vi "RSZVB Get Remote Display Title.vi"(8 "error in (no error)":errorcluster {"code" format="%.0x"}, 11 "VISA session":refnum<visa-resource-name>) -> (0 "error out":errorcluster {"code" format="%.0x"}, 1 "Title":string, 3 "dup VISA session":refnum<visa-resource-name>)   [LabVIEW 2011]
doc: "This function queries title for the remote display.\n\nRemote-control command(s):\nSYSTem:USER:DISPlay:TITLe?"
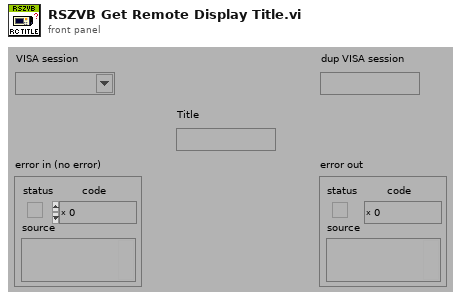
[diagram p1: front panel]
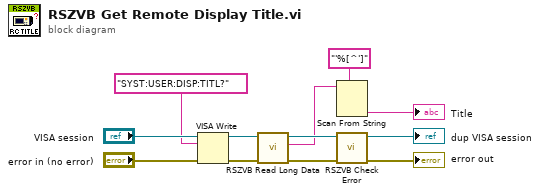
[diagram p0: block diagram]
diagram:
  n1 = VISA Write(VISA resource name="VISA session", write buffer="SYST:USER:DISP:TITL?", error in (no error)="error in (no error)") -> (VISA resource name out=w5:refnum<visa-resource-name>, error out=w4:errorcluster)  [unwired: 1 out]
  n2 = call "RSZVB Read Long Data.vi"("error in (no error)"=w4, "VISA resource name"=w5) -> ("error out"=w1:errorcluster, "Data"=w2:string, "VISA resource name out"=w3:refnum<visa-resource-name>)  [unwired: 7 in]
  n3 = Scan From String(format string="'%[^']", input string=w2) -> (output 1=→"Title":string)  [unwired: 3 in, 3 out]
  n4 = call "RSZVB Check Error.vi"("error in (no error)"=w1, "VISA session"=w3) -> ("error out"=→"error out":errorcluster, "dup VISA session"=→"dup VISA session":refnum<visa-resource-name>)  [unwired: 8 in]
